vi "LeCroy Wave Series Acquire Timed Sequence.vi"() -> ()   [LabVIEW 2018]
doc: "This example configures the sequence acquisition mode, initiates the acquisition, waits for the acquisition to complete and reads all acquired segments. The segment data contain timestamping information.\n\nNote:\n\nSequence Acquisitions are not supported by WaveSurfer models."
uses:
  LeCroy Wave Series.lvlib
panel:
  in  "Number of Segments (2)":u16=2
  in  "Source (0: Channel 1)":u16(ring) items=["Channel 1", "Channel 2", "Channel 3", "Channel 4", "Memory 1", "Memory 2", "Memory 3", "Memory 4", "Function 1", "Function 2", "Function 3", "Function 4", "Function 5", "Function 6", "Function 7", "Function 8"]
  out "Waveform Data":waveform(dbl)[](graph)
  in  "Timeout (10000 ms)":u32=10000
  in  "VISA resource name":refnum<visa-resource-name>="waveRunner6100"
  # "(c) 2005 - 2012 NATIONAL INSTRUMENTS.  ALL RIGHTS RESERVED."
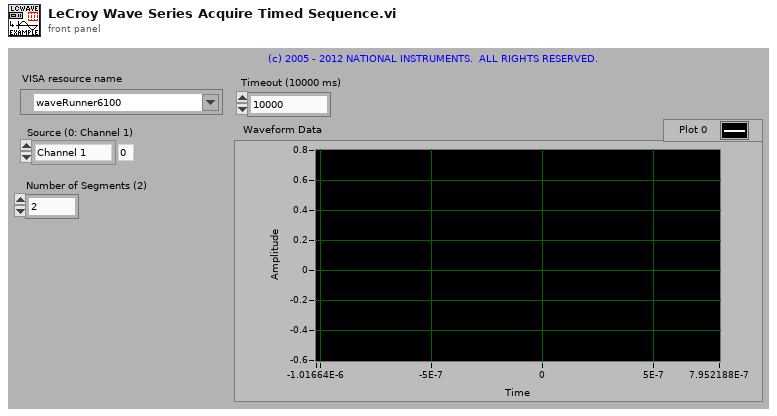
[diagram p1: front panel]
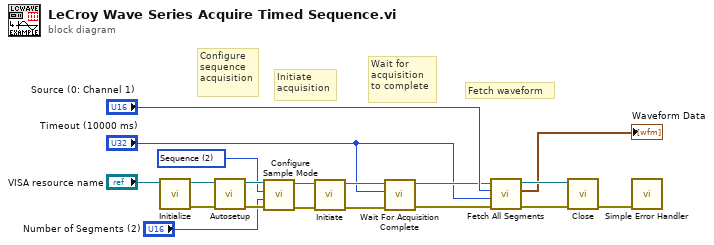
[diagram p0: block diagram]
diagram:
  w1 = u16 2 items=["RealTime", "RIS", "Sequence", "Roll", "WaveStream"] ("Sample Mode (0: RealTime)")
  # "Fetch waveform"
  # "Wait for \nacquisition\nto complete"
  # "Initiate\nacquisition"
  # "Configure sequence\nacquisition"
  n1 = call "Initialize.vi"("VISA resource name"="VISA resource name") -> ("error out"=w6:errorcluster, "VISA resource name out"=w7:refnum<visa-resource-name>)  [unwired: 9 in]
  n2 = call "Autosetup.vi"("error in (no error)"=w6, "VISA resource name"=w7) -> ("error out"=w4:errorcluster, "VISA resource name out"=w5:refnum<visa-resource-name>)  [unwired: 8 in]
  n3 = call "Configure Sample Mode.vi"("error in (no error)"=w4, "Number of Segments (2)"="Number of Segments (2)", "Sample Mode (0: RealTime)"=w1, "VISA resource name"=w5) -> ("error out"=w12:errorcluster, "VISA resource name out"=w13:refnum<visa-resource-name>)  [unwired: 6 in]
  n4 = call "Initiate.vi"("error in (no error)"=w12, "VISA resource name"=w13) -> ("error out"=w8:errorcluster, "VISA resource name out"=w11:refnum<visa-resource-name>)  [unwired: 8 in]
  n5 = call "Wait For Acquisition Complete.vi"("error in (no error)"=w8, "Timeout (10000 ms)"="Timeout (10000 ms)", "VISA resource name"=w11) -> ("error out"=w9:errorcluster, "VISA resource name out"=w10:refnum<visa-resource-name>)  [unwired: 6 in, 1 out]
  n6 = call "Fetch All Segments.vi"("error in (no error)"=w9, "Timeout (10000 ms)"="Timeout (10000 ms)", "Source (0: Channel 1)"="Source (0: Channel 1)", "VISA resource name"=w10) -> ("error out"=w17:errorcluster, "Array"=→"Waveform Data":waveform(dbl)[], "VISA resource name out"=w18:refnum<visa-resource-name>)  [unwired: 5 in]
  n7 = call "Close.vi"("error in (no error)"=w17, "VISA resource name"=w18) -> ("error out"=w19:errorcluster)  [unwired: 9 in]
  n8 = call <vilib>:"Simple Error Handler.vi"("error in (no error)"=w19) -> ()  [unwired: 4 in, 5 out]
